vi "Read Config from File.vi"(6 "Comment out unparsable lines":bool=TRUE, 7 "Template (JSON Object)":string="// JSONtext Config File\n{}", 8 "error in (no error)":errorcluster, 10 "config file path":path) -> (0 "error out":errorcluster, 1 "Template Used (file missing or corrupted)":bool, 2 "<JSON>Config":string, 3 "Config File":refnum<class "Config File.lvclass">)   [LabVIEW 2020, in "Config File.lvclass"]
doc: "Read in the Configuration from the specified file. If the file does not exists, a supplied Template will be used (if input). The Template should be a JSON Object and may include Comments."
uses:
  <vilib>/JDP Science/JSONtext/Config Files/Config File.lvclass
  <vilib>/JDP Science/JSONtext/Config Files/Config File.lvclass/Config File.ctl
  <vilib>/JDP Science/JSONtext/support/Format Error.vi
  <vilib>/JDP Science/JSONtext/JSON type.vi
  <vilib>/Utility/error.llb/Error Cluster From Error Code.vi
  <vilib>/JDP Science/JSONtext/JSONtext.lvlib
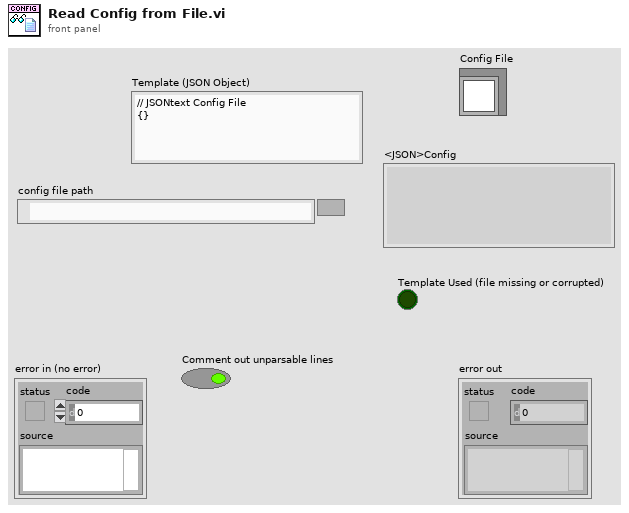
[diagram p1: front panel]
types:
  T1 = enum16{"open", "replace", "create", "open or create", "replace or create", "replace or create with confirmation"}
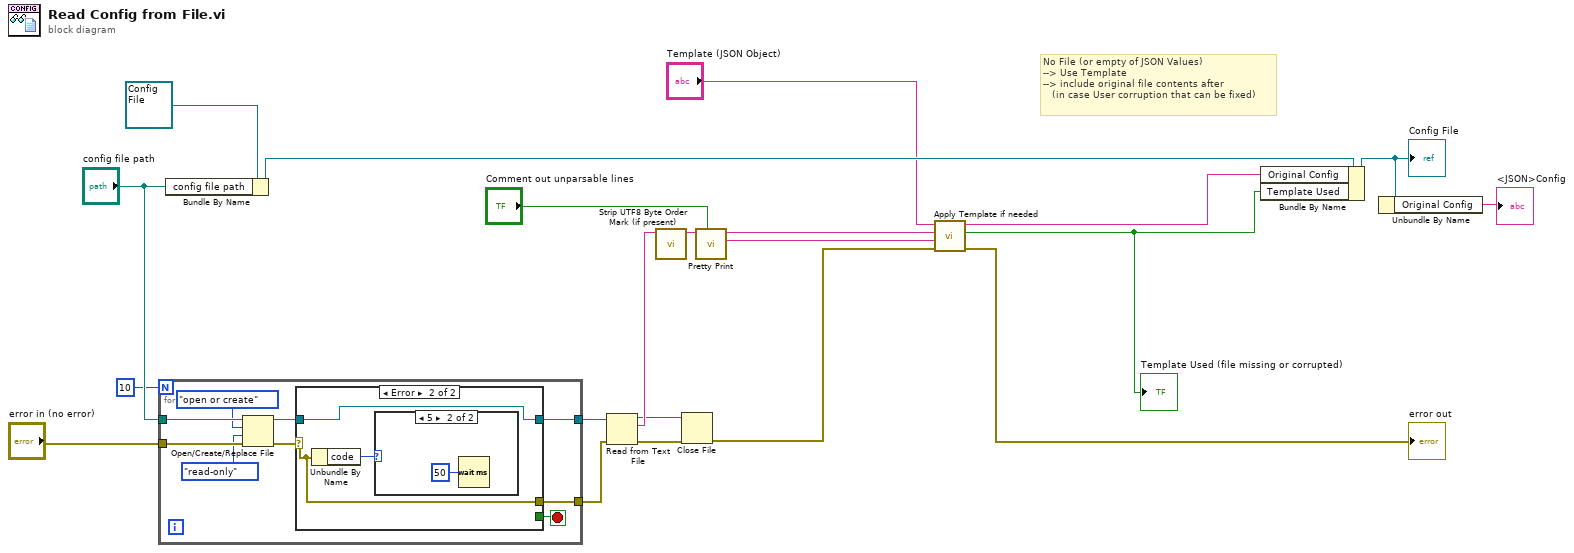
[diagram p0: block diagram]
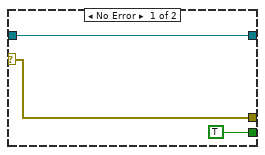
[diagram p2: hidden frame]
diagram:
  # "No File (or empty of JSON Values)\n--> Use Template\n--> include original file contents after\n   (in case User corruption that can be fixed)"
  n1 = for {
    N: 10 -> [_]
    tunnel: "config file path" -> [w30]
    tunnel: [w27] -> w3
    tunnel: "error in (no error)" -> [w25]
    tunnel: [w24] -> w2
    stop <- w26 stop-if-true
    n2 = Open/Create/Replace File(file path (use dialog)=w30, error in=w25, operation (0:open)=T1."open or create", access (0:read/write)=enum16{"read/write", "read-only", "write-only"}."read-only") -> (refnum out=w28:refnum<file>, error out=w29:errorcluster)  [unwired: 2 in, 1 out]
    n3 = case shown="Error" w29 {
      selector: w29 -> [w31 w34]
      tunnel: w28 -> [w33 w35]
      tunnel: [w33 w35] -> w27
      tunnel: [TRUE _] -> w26
      tunnel: [w31 w34] -> w24
      frame No Error {
      }
      frame Error {
        n4 = Unbundle By Name(w34) -> ("code"=w36:i32)
        n5 = case shown="5" w36 {
          frame 0, Default {
          }
          frame 5 {
            n6 = Wait (ms)(milliseconds to wait=u32 50) -> ()  [unwired: 1 out]
          }
        }
      }
    }
  }
  n7 = Bundle By Name(cluster=refnum<class "Config File.lvclass"> refnum ("Config File in"), "config file path"="config file path") -> (w20:refnum<class "Config File.lvclass">)
  n8 = Read from Text File(file (use dialog)=w3, error in=w2) -> (refnum out=w16:refnum<file>, text=w19:string, error out=w17:errorcluster)  [unwired: 2 in, 1 out]
  n9 = call <vilib>:"Strip UTF8 Byte Order Mark (if present).vi"("Text in"=w19) -> ("Possible Byte Order Mark Stripped"=w18:string)  [unwired: 9 in, 1 out]
  n10 = Close File(refnum=w16, error in=w17) -> (error out=w8:errorcluster)  [unwired: 1 out]
  n11 = call <vilib>:"Pretty Print.vi"("Comment out unparsable lines"="Comment out unparsable lines", "JSON"=w18) -> ("Rest of Input String"=w9:string, "<JSON>"=w12:string)  [unwired: 7 in, 1 out]
  n12 = call <vilib>:"Apply Template if needed.vi"("error in (no error)"=w8, "Rest of Input String"=w9, "From File"=w12, "Template"="Template (JSON Object)") -> ("error out"=→"error out":errorcluster, "Template Applied"=w6:bool, "<JSON>"=w11:string)  [unwired: 5 in]
  "Template Used (file missing or corrupted)" <- w6
  n13 = Bundle By Name(cluster=w20, "Original Config"=w11, "Template Used"=w6) -> (w14:refnum<class "Config File.lvclass">)
  "Config File" <- w14
  n14 = Unbundle By Name(w14) -> ("Original Config"=→"<JSON>Config":string)
